vi "Initialize Values.vi"(8 "error in (no error)":errorcluster, 11 "Mastering in":refnum<class "Mastering.lvclass">) -> (0 "error out":errorcluster, 3 "Mastering out":refnum<class "Mastering.lvclass">)   [LabVIEW 2014, in "SeqLoop.lvlib" / "STEP Classes.lvlib" / "Mastering.lvclass"]
uses:
  Mastering.lvclass
  Mastering.lvclass/Mastering.ctl
  STEP/STEP.lvclass
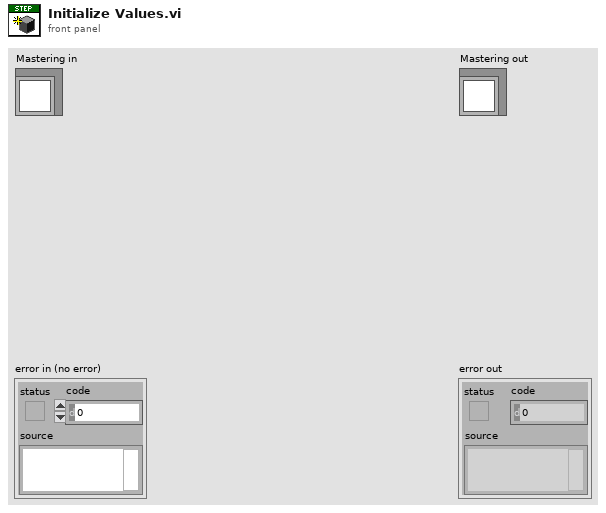
[diagram p1: front panel]
types:
  T1 = cluster{"HWSync 1":bool, "HWSync 2":bool, "HWSync 3":bool, "HWSync 4":bool, "HWSync 5":bool}
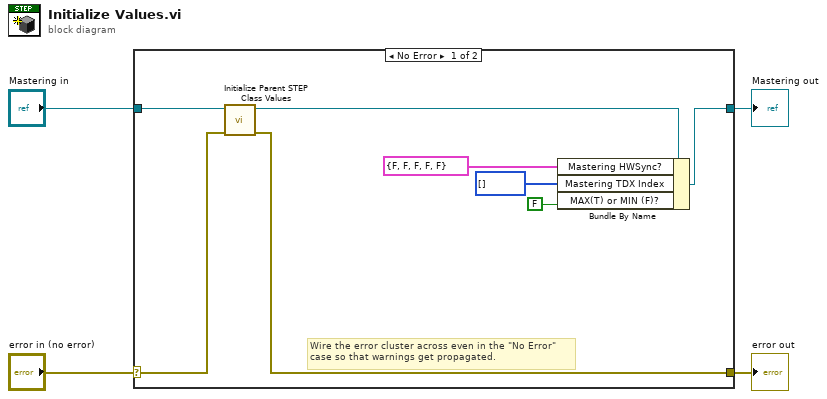
[diagram p0: block diagram]
diagram:
  n1 = case shown="No Error" "error in (no error)" {
    selector: "error in (no error)" -> [w12 w14]
    tunnel: [w11 w14] -> w3
    tunnel: [w8 w13] -> w1
    tunnel: "Mastering in" -> [w10 w13]
    frame No Error {
      # "Wire the error cluster across even in the \"No Error\"\ncase so that warnings get propagated."
      n2 = call "Initialize Parent STEP Class Values.vi"("error in (no error)"=w12, "STEP in"=w10) -> ("error out"=w11:errorcluster, "STEP out"=w9:refnum<class "Mastering.lvclass">)  [unwired: 8 in]
      n3 = Bundle By Name(cluster=w9, "Mastering HWSync?"=T1 {"HWSync 1"=FALSE, "HWSync 2"=FALSE, "HWSync 3"=FALSE, "HWSync 4"=FALSE, "HWSync 5"=FALSE}, "Mastering TDX Index"=i32[] [], "MAX(T) or MIN (F)?"=FALSE) -> (w8:refnum<class "Mastering.lvclass">)
    }
    frame Error {
    }
  }
  "error out" <- w3
  "Mastering out" <- w1
